vi "Shooter Loop.vi"   [LabVIEW 2015]
uses:
  Common Code/Shooter State.ctl
  Robot Global Data.vi
types:
  T1 = typedef "WPI_DigitalInputDevRef.ctl" = cluster{"DevStatus":errorcluster, "DIO Channel":T2}
  T2 = typedef "FPGA_DIOChannel.ctl" = enum8{"DIO 0", "DIO 1", "DIO 2", "DIO 3", "DIO 4", "DIO 5", "DIO 6", "DIO 7", "DIO 8", "DIO 9", "DIO MXP 0", "DIO MXP 1", "DIO MXP 2", "DIO MXP 3", "DIO MXP 4", "DIO MXP 5", "DIO MXP 6", "DIO MXP 7", "DIO MXP 8", "DIO MXP 9", "DIO MXP 10", "DIO MXP 11", "DIO MXP 12", "DIO MXP 13", "DIO MXP 14", "DIO MXP 15", "Invalid"}
  T3 = typedef "Shooter Command Cluster.ctl" = cluster{"Command":T4, "Mode":T5, "Shot Type":T6, "Override Trigger Sensor":bool, "Override Angle?":bool, "Hide From Death":bool}
  T4 = typedef "Shooter Commands.ctl" = enum16{"Idle", "Prime Shooter", "Shoot"}
  T5 = typedef "Shoot Modes Enum.ctl" = enum16{"Manual", "Safe", "Auto"}
  T6 = typedef "Shot Type.ctl" = enum16{"Batter Shot", "Corner Shot", "Cleat Shot", "Vision Shot", "Deep Middle Shot"}
  T7 = typedef "Manual Shoot.ctl" = cluster{"Spin Wheels":bool, "Fire":bool, "Angle":dbl, "Angle Power":dbl, "Use Manual Angle":bool, "Override RPM":bool, "Left RPM":dbl, "Right RPM":dbl, "Secure Ball?":bool}
  T8 = typedef "Shooter State.ctl" = enum16{"Idle", "Warmup", "Shooter Ready", "Shoot"}
  T9 = typedef "Dashboard Control Data.ctl" = cluster{"Shooter Presets":T10, "Encoder Control":T12, "Steer PID output":cluster{"output high":dbl, "output low":dbl}, " Steer PID gains":cluster{"proportional gain (Kc)":dbl, "integral time (Ti, min)":dbl, "derivative time (Td, min)":dbl}, "Drivetrain Settings":T13, "Vision Packet":T14, "Dashboard Drivetrain Command":T15, "Info/Command Cluster":T17, "Ball Vision Packet":T18, "Intake Presets":T20, "Intake Encoder Control":T22, "Climb Presets":T23, "Goal Output Range":cluster{"output high":dbl, "output low":dbl}, "Enabled Systems":T24, "Auton Presets":T25, "Pressure M":dbl, "Pressure B":dbl}
  T10 = typedef "Shooter Presets.ctl" = cluster{"Batter Shot":T11, "Deep Middle":T11, "Manual Shot":T11, "Left Ticks Per Rotation":dbl, "Right Ticks Per Rotation":dbl, "Low Bar Shot":T11, "Shooter RPM Tolerance":dbl, "Trigger Power":dbl, "Fire from Load Delay":i32, "Max Angle":dbl, "Min Angle":dbl, "Angle PID gains":cluster{"P":dbl, "I":dbl, "D":dbl}, "Angle Output":cluster{"output high":dbl, "output low":dbl}, "Shooter Angle Tolerance":dbl, "Vision Shoot x^2":dbl, "Vision Shoot x":dbl, "Feed Forward Max Accel":dbl, "Feed Forward Kv":dbl, "Backwards Trigger":dbl, "Shot Finish Delay (ms)":dbl, "Angle Max Current":dbl, "Angle Current Trip Time":dbl, "Intake Angle":dbl, "Vision Shoot c":dbl, "Reset?":bool, "Button Release Delay":dbl, "Angle Pot x":dbl, "Angle Pot c":dbl, "Ignore Angle?":bool, "Max RPM":dbl, "Safty Frist Angle":dbl, "Intake Danger Height":dbl, "Angle Pot B":i32, "Angle Pot M":dbl, "FF Finish RPM":dbl, "RPM PID Right":cluster{"P":dbl, "I":dbl, "D":dbl, "FF":dbl}, "RPM PID Left":cluster{"P":dbl, "I":dbl, "D":dbl, "FF":dbl}, "Backwards RPM":dbl, "Vision RPM":dbl, "Run Wheels Backward Delay":u32, "Cleat Shot":T11}
  T11 = typedef "Shot Presets.ctl" = cluster{"L":dbl, "R":dbl, "A":dbl}
  T12 = typedef "Encoder Control.ctl" = cluster{"Right Tick Constant":dbl, "Left Tick Constant":dbl, "Reset?":bool, "Y Dist":cluster{"PID gains":cluster{"proportional gain (Kc)":dbl, "integral time (Ti, min)":dbl, "derivative time (Td, min)":dbl}}, "Y Stop Thresh":dbl, "Y Stop Speed":dbl}
  T13 = typedef "Drivetrain Settings.ctl" = cluster{"Gyro Tolerance":dbl, "Throttle Ramp (ms)":dbl, "Kv":dbl, "Ka":dbl, "Feed Forward P":dbl, "Feed Forward D":dbl, "Goal Vision PID gains":cluster{"proportional gain (Kc)":dbl, "integral time (Ti, min)":dbl, "derivative time (Td, min)":dbl}, "Goal Detection Window":dbl, "Creep Rate":dbl, "Vision Throttle Threshold":dbl, "Min Turn Output":dbl, "Left Batter Angle":dbl, "Right Batter Angle":dbl}
  T14 = typedef "Goal Vision Packet.ctl" = cluster{"Distance":dbl, "Center X":dbl, "Center Y":dbl, "Found Target?":bool, "Robot Center":dbl, "Angle":dbl}
  T15 = typedef "Dashboard Drivetrain Command.ctl" = cluster{"Drivetrain Vision":T16}
  T16 = typedef "Drivetrain Vision.ctl" = cluster{"Goal Window":dbl, "Ball Window":dbl}
  T17 = typedef "Ball Tracking Command Cluster.ctl" = cluster{"Distance to Ball":dbl, "Desired Angle":dbl, "Command":enum16{"Turn to Ball", "Turn to Angle", "Get Distance"}, "Pixels from Center":dbl}
  T18 = typedef "Ball Vision Packet.ctl" = cluster{"Ball Detected?":bool, "Distance to Ball":dbl, "Desired Angle":dbl, "Pixels from Center":dbl, "Tracking mode":T19}
  T19 = typedef "Tracking Mode.ctl" = enum16{"Turn to Ball", "Turn to Angle"}
  T20 = typedef "Intake Presets.ctl" = cluster{"Intake Speed":dbl, "Outake Speed":dbl, "Low Height":dbl, "Half Height":dbl, "Full Height":dbl, "Angle Speed":dbl, "Angle Tolerance":dbl, "Encoder Scale":dbl, "Load Height":dbl, "Output Range":T21, "Rotation Power Max/Min":dbl, "MaxCurrent":dbl, "Intake Trip Time":dbl, "Idle Height":dbl, "Max Height":dbl, "Reset Encoders?":bool, "PID gains":cluster{"proportional gain (Kc)":dbl, "integral time (Ti, min)":dbl, "derivative time (Td, min)":dbl}, "Intake Stop Delay":u32, "Settle Time":dbl, "Settle Wait Time":dbl}
  T21 = typedef "Drivetrain Output Range.ctl" = cluster{"output high":dbl, "output low":dbl}
  T22 = typedef "IntakeEcoderControl.ctl" = cluster{"Arm Tick Constant":dbl, "Reset?":bool, "Y Dist":cluster{"PID gains":cluster{"proportional gain (Kc)":dbl, "integral time (Ti, min)":dbl, "derivative time (Td, min)":dbl}}, "Y Stop Thresh":dbl, "Y Stop Speed":dbl}
  T23 = typedef "Climb Presets.ctl" = cluster{"Pull Power":dbl, "Extend Power":dbl}
  T24 = typedef "Enabled Systems.ctl" = cluster{"Shoot":bool, "Intake":bool, "DT":bool, "Gyro":bool, "100ms":bool, "US":bool}
  T25 = typedef "Autonomous Presets.ctl" = cluster{"Pitch Limit":dbl, "Roll Limit":dbl, "Start Position":dbl, "Cross Position":dbl}
  T26 = typedef "WPI_ServoDeviceRef.ctl" = cluster{"DeviceStatus":errorcluster, "PWM Channel":T27, "DeadBand":T28}
  T27 = typedef "FPGA_DIOPWMChannel.ctl" = enum8{"PWM 0", "PWM 1", "PWM 2", "PWM 3", "PWM 4", "PWM 5", "PWM 6", "PWM 7", "PWM 8", "PWM 9", "PWM MXP 0", "PWM MXP 1", "PWM MXP 2", "PWM MXP 3", "PWM MXP 4", "PWM MXP 5", "PWM MXP 6", "PWM MXP 7", "PWM MXP 8", "PWM MXP 9", "Invalid"}
  T28 = typedef "WPI_PWMDeadband.ctl" = cluster{"Name":string, "maxPositivePwm":i32, "minPositivePwm":i32, "centerPwm":i32, "maxNegativePwm":i32, "minNegativePwm":i32, "angularRange":u16}
  T29 = typedef "WPI_MotorControlDeviceRef.ctl" = cluster{"DeviceStatus":errorcluster, "Type":T30, "PWM":cluster{"PWM Channel":T27, "DeadBand":T28}, "CAN":cluster{"Device Number":u8, "Control Mode":T31, "Semaphore":T32, "Max Vout":dbl, "TalonSRX Control Mode":T33}, "Invert":bool}
  T30 = typedef "WPI_MotorControlType.ctl" = enum16{"PWM", "CAN", "CANTalonSRX"}
  T31 = typedef "WPI_CANJaguar_ControlMode.ctl" = enum8{"Percent VBus", "Current", "Speed", "Position", "Voltage"}
  T32 = typedef "Semaphore RefNum" = refnum<k1>
  T33 = typedef "WPI_CANTalonSRX_APIControlMode.ctl" = enum8{"Percent VBus", "Speed", "Position", "Slave", "Unchanged / Invalid", "Voltage Compensation", "Current", "Motion Profile"}
  T34 = typedef "Shooter State Cluster.ctl" = cluster{"State":T8, "Left RPM":dbl, "Right RPM":dbl, "Shooter Ready?":bool, "Ball Loaded?":bool, "Current Angle":dbl, "Angle Motor Output":dbl, "Trigger Output":dbl, "Angle Ready?":bool, "RPM Ready?":bool, "Vision Ready?":bool, "Ball Loaded?":bool, "Mode":T5, "Shot Type":T6, "Pot Height":dbl, "Current Tripped Forward?":bool, "Current Tripped Backward?":bool, "Right Servo":i32, "Left Servo":i32, "IR Override":bool, "Intake Danger?":bool, "Intake Angle Ready?":bool}
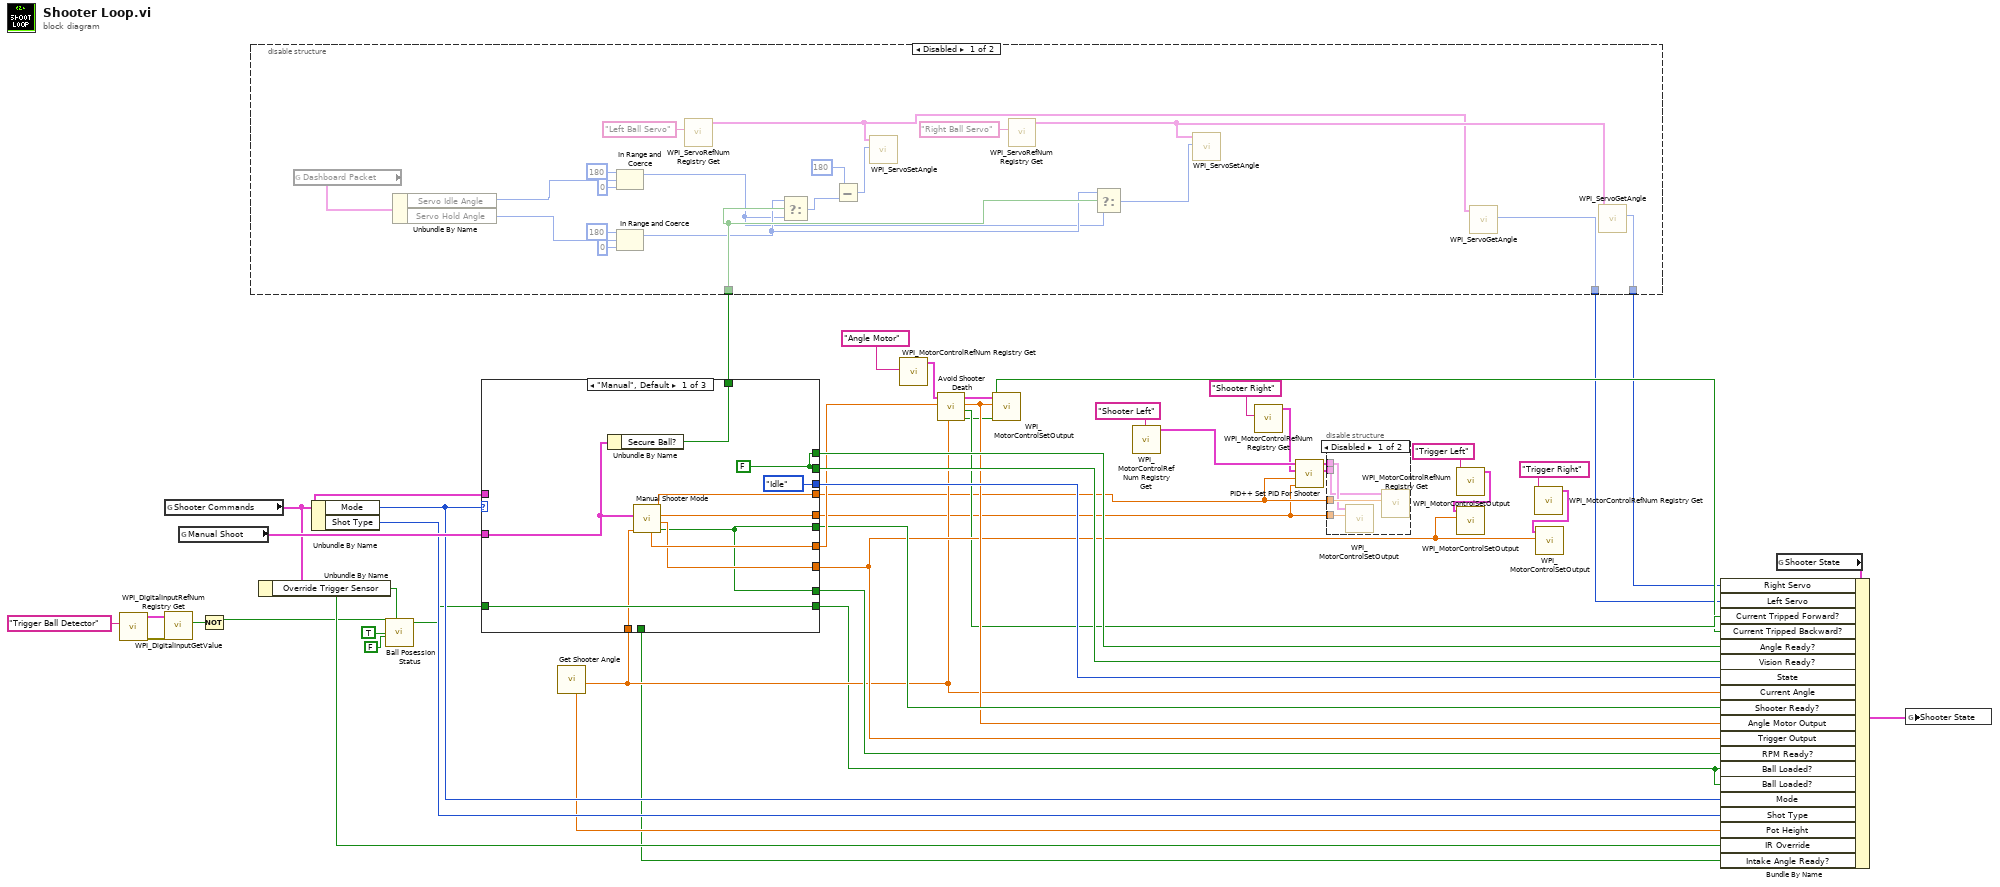
[diagram p0: block diagram]
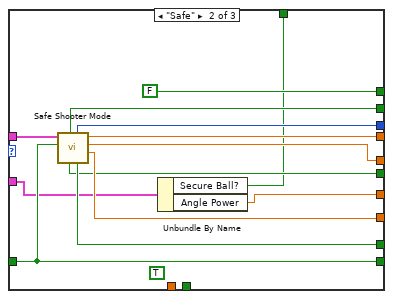
[diagram p4: hidden frame]
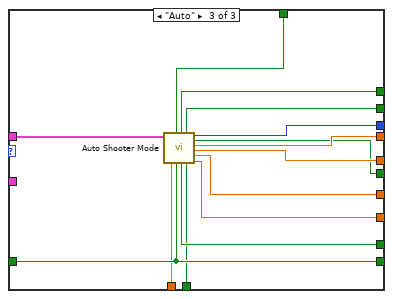
[diagram p5: hidden frame]
diagram:
  n1 = call <vilib>:"WPI_DigitalInputRefNum Registry Get.vi"("refnum name"="Trigger Ball Detector") -> ("error out"=w10:errorcluster, "DigitalInputDevRef"=w9:T1)  [unwired: 9 in]
  n2 = global read "Robot Global Data.vi" "Shooter Commands"() -> (w44:T3)
  n3 = call <vilib>:"WPI_DigitalInputGetValue.vi"("error in (no error)"=w10, "DigitalInputDevRef"=w9) -> ("Value"=w4:bool)  [unwired: 7 in, 2 out]
  n4 = global read "Robot Global Data.vi" "Manual Shoot"() -> (w45:T7)
  n5 = Not(x=w4) -> (.not. x?=w3:bool)
  n6 = Unbundle By Name(w44) -> ("Override Trigger Sensor"=w13:bool)
  n7 = Unbundle By Name(w44) -> ("Mode"=w39:T5, "Shot Type"=w38:T6)
  n8 = call "Ball Posession Status.vi"("Override?"=w13, "Logical Exit?"=FALSE, "Using Sensor?"=TRUE, "Sensor"=w3) -> ("Ball Posessed?"=w12:bool)  [unwired: 7 in]
  n9 = call "Get Shooter Angle.vi"() -> ("Current Angle"=w27:dbl, "Pot Height"=w28:dbl)  [unwired: 10 in]
  n10 = case shown="\"Manual\", Default" w39 {
    tunnel: w44 -> [_ w71 w85]
    tunnel: w45 -> [w50 w62 _]
    tunnel: [w58 w69 w79] -> w2
    tunnel: [w55 w68 w80] -> w1
    tunnel: [w53 w63 w75] -> w36
    tunnel: w12 -> [w57 w70 w84]
    tunnel: [w57 w70 w84] -> w7
    tunnel: [w56 w61 w81] -> w37
    tunnel: [w54 w67 w82] -> w34
    tunnel: [w53 w65 w83] -> w42
    tunnel: [Shooter_State."Idle" ("State") w66 w78] -> w43
    tunnel: [w51 w64 w77] -> w40
    tunnel: [w51 FALSE ("Angle In Range?") w76] -> w41
    tunnel: [w49 w59 w74] -> w31
    tunnel: w27 -> [w48 _ w73]
    tunnel: [_ _ w72] -> w5
    frame "Manual", Default {
      w51 = FALSE ("Vision Target Aligned?")
      n11 = Unbundle By Name(w50) -> ("Secure Ball?"=w49:bool)
      n12 = call "Manual Shooter Mode.vi"("Shooter Angle"=w48, "Manual Shoot"=w50) -> ("Shooter Ready?"=w53:bool, "Trigger Output"=w54:dbl, "Right Output"=w55:dbl, "Left Output"=w58:dbl, "Angle Motor Out"=w56:dbl)  [unwired: 5 in]
    }
    frame "Safe" {
      (unwired) TRUE ("Intake High Angle Allowed?")
      n13 = call "Safe Shooter Mode.vi"("Ball Detected?"=w70, "Shooter Commands"=w71) -> ("Trigger Power"=w67:dbl, "Right Power"=w68:dbl, "Left Power"=w69:dbl, "RPM Ready?"=w65:bool, "State"=w66:T8, "Shooter Ready?"=w63:bool, "Vision Ready?"=w64:bool)  [unwired: 3 in]
      n14 = Unbundle By Name(w62) -> ("Secure Ball?"=w59:bool, "Angle Power"=w61:dbl)
    }
    frame "Auto" {
      n15 = call "Auto Shooter Mode.vi"("Shooter Command"=w85, "Current Angle"=w73, "Ball Loaded?"=w84) -> ("Secure Ball?"=w74:bool, "Angle In Range?"=w76:bool, "RPM Ready?"=w83:bool, "Vision Target Aligned?"=w77:bool, "Intake Ready?"=w72:bool, "State"=w78:T8, "Shooter Ready?"=w75:bool, "Left Output"=w79:dbl, "Right Output"=w80:dbl, "Angle Motor Output"=w81:dbl, "Trigger Output"=w82:dbl)  [unwired: 6 in]
    }
  }
  n16 = disable-structure shown="Disabled" {
    disable-tunnel: w31 -> [w105 _]
    disable-tunnel: [w104 _] -> w30
    disable-tunnel: [w103 _] -> w29
    frame Disabled {
      n17 = global read "Robot Global Data.vi" "Dashboard Packet"() -> (w100:T9)
      n18 = Unbundle By Name(w100) -> ("Servo Idle Angle"=w96:i32, "Servo Hold Angle"=w91:i32)
      n19 = In Range and Coerce(upper limit=180, x=w96, lower limit=0) -> (coerced(x)=w89:i32)  [unwired: 1 out]
      n20 = In Range and Coerce(upper limit=180, x=w91, lower limit=0) -> (coerced(x)=w90:i32)  [unwired: 1 out]
      n21 = call <vilib>:"WPI_ServoRefNum Registry Get.vi"("refnum name"="Left Ball Servo") -> ("ServoDeviceRef"=w97:T26)  [unwired: 9 in, 1 out]
      n22 = Select(t=w90, s=w105, f=w89) -> (s? t:f=w87:i32)
      n23 = Subtract(x=180, y=w87) -> (x-y=w86:i32)
      n24 = call <vilib>:"WPI_ServoSetAngle.vi"("Angle"=w86, "ServoDeviceRef"=w97) -> ()  [unwired: 8 in, 2 out]
      n25 = call <vilib>:"WPI_ServoRefNum Registry Get.vi"("refnum name"="Right Ball Servo") -> ("ServoDeviceRef"=w99:T26)  [unwired: 9 in, 1 out]
      n26 = Select(t=w90, s=w105, f=w89) -> (s? t:f=w98:i32)
      n27 = call <vilib>:"WPI_ServoSetAngle.vi"("Angle"=w98, "ServoDeviceRef"=w99) -> ()  [unwired: 8 in, 2 out]
      n28 = call <vilib>:"WPI_ServoGetAngle.vi"("ServoDeviceRef"=w97) -> ("Angle"=w103:u16)  [unwired: 7 in, 2 out]
      n29 = call <vilib>:"WPI_ServoGetAngle.vi"("ServoDeviceRef"=w99) -> ("Angle"=w104:u16)  [unwired: 7 in, 2 out]
    }
    frame Enabled {
    }
  }
  n30 = call <vilib>:"WPI_MotorControlRefNum Registry Get.vi"("refnum name"="Angle Motor") -> ("MotorControlDevRef"=w25:T29)  [unwired: 9 in, 1 out]
  n31 = call "Avoid Shooter Death.vi"("Shooter Angle"=w27, "Proposed Power"=w37, "CAN Talon SRX Ref"=w25) -> ("Reverse Trip?"=w32:bool, "Forward Trip?"=w33:bool, "Actual Output"=w35:dbl, "CAN Talon SRX Ref 2"=w24:T29)  [unwired: 5 in]
  n32 = call <vilib>:"WPI_MotorControlSetOutput.vi"("Output"=w35, "MotorControlDevRef"=w24) -> ()  [unwired: 7 in, 3 out]
  n33 = call <vilib>:"WPI_MotorControlRefNum Registry Get.vi"("refnum name"="Shooter Left") -> ("MotorControlDevRef"=w17:T29)  [unwired: 9 in, 1 out]
  n34 = call <vilib>:"WPI_MotorControlRefNum Registry Get.vi"("refnum name"="Shooter Right") -> ("MotorControlDevRef"=w16:T29)  [unwired: 9 in, 1 out]
  n35 = call "PID++ Set PID For Shooter.vi"("Shooter Right"=w1, "Shooter Left"=w2, "Right Shooter Motor"=w16, "Left Shooter Motor"=w17) -> ("Right Shooter Motor Out"=w14:T29, "Left Shooter Motor Out"=w15:T29)  [unwired: 6 in]
  n36 = disable-structure shown="Disabled" {
    disable-tunnel: w2 -> [w109 _]
    disable-tunnel: w1 -> [w108 _]
    disable-tunnel: w15 -> [w107 _]
    disable-tunnel: w14 -> [w106 _]
    frame Disabled {
      n37 = call <vilib>:"WPI_MotorControlSetOutput.vi"("Output"=w108, "MotorControlDevRef"=w107) -> ()  [unwired: 7 in, 3 out]
      n38 = call <vilib>:"WPI_MotorControlSetOutput.vi"("Output"=w109, "MotorControlDevRef"=w106) -> ()  [unwired: 7 in, 3 out]
    }
    frame Enabled {
    }
  }
  n39 = call <vilib>:"WPI_MotorControlRefNum Registry Get.vi"("refnum name"="Trigger Left") -> ("MotorControlDevRef"=w21:T29)  [unwired: 9 in, 1 out]
  n40 = call <vilib>:"WPI_MotorControlSetOutput.vi"("Output"=w34, "MotorControlDevRef"=w21) -> ()  [unwired: 7 in, 3 out]
  n41 = call <vilib>:"WPI_MotorControlRefNum Registry Get.vi"("refnum name"="Trigger Right") -> ("MotorControlDevRef"=w20:T29)  [unwired: 9 in, 1 out]
  n42 = call <vilib>:"WPI_MotorControlSetOutput.vi"("Output"=w34, "MotorControlDevRef"=w20) -> ()  [unwired: 7 in, 3 out]
  n43 = global read "Robot Global Data.vi" "Shooter State"() -> (w47:T34)
  n44 = Bundle By Name(cluster=w47, "Right Servo"=w30, "Left Servo"=w29, "Current Tripped Forward?"=w33, "Current Tripped Backward?"=w32, "Angle Ready?"=w41, "Vision Ready?"=w40, "State"=w43, "Current Angle"=w27, "Shooter Ready?"=w36, "Angle Motor Output"=w35, "Trigger Output"=w34, "RPM Ready?"=w42, "Ball Loaded?"=w7, "Ball Loaded?"=w7, "Mode"=w39, "Shot Type"=w38, "Pot Height"=w28, "IR Override"=w13, "Intake Angle Ready?"=w5) -> (w46:T34)
  n45 = global write "Robot Global Data.vi" "Shooter State"(w46) -> ()
